vi "Jaguar Commands.vi"() -> ()   [LabVIEW 2012]
panel:
  in  "Actuator Volt Limit":dbl=0.4
  in  "Gatherer":dbl
  in  "Actuator":dbl=2.0421915555
  in  "Shooters":dbl
  in  "Rear Right Steer":dbl=3.10886
  in  "Rear Left Steer":dbl=1.557035
  in  "Front Right Steer":dbl=1.2732370000000002
  in  "Front Left Steer":dbl=2.79833
  in  "Rear Right Drive":dbl=-0.0
  in  "Rear Left Drive":dbl
  in  "Front Right Drive":dbl=-0.0
  in  "Front Left Drive":dbl
  # "Drives"
  # "Steers"
  # "Miscellaneous"
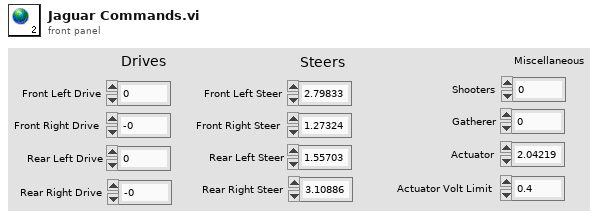
[diagram p1: front panel]
diagram:
